vi "GetProperties.vi"(8 "error in":errorcluster, 11 "Decoration in":refnum<class "Decoration.lvclass">) -> (0 "error out":errorcluster, 3 "Decoration out":refnum<class "Decoration.lvclass">)   [LabVIEW 2014, in "Raspberry Pi Compatible Compiler for LabVIEW.lvlib" / "Decoration.lvclass"]
uses:
  Decoration.lvclass
  Decoration.lvclass/Decoration.ctl
  GObject/GObject.lvclass
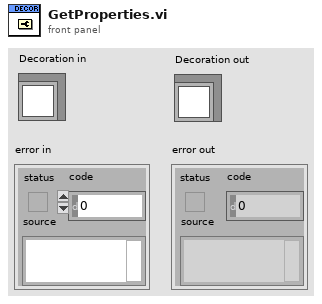
[diagram p1: front panel]
types:
  T1 = typedef "LVForegroundBackgroundColorsTypeDef.ctl" = cluster{"FG Color":u32, "BG Color":u32}
  T2 = typedef "LVBoundsTypeDef.ctl" = cluster{"Width":u32, "Height":u32}
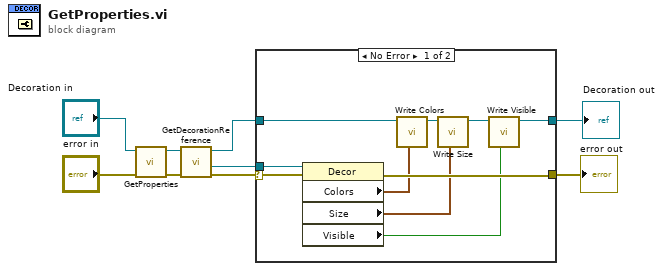
[diagram p0: block diagram]
diagram:
  n1 = call-parent "GetProperties.vi"("error in"="error in", "GObject in"="Decoration in") -> ("error out"=w2:errorcluster, "GObject out"=w4:refnum<class "Decoration.lvclass">)  [unwired: 8 in]
  n2 = call "GetDecorationReference.vi"("error in"=w2, "Decoration in"=w4) -> ("error out"=w6:errorcluster, "Decoration reference"=w5:refnum<vi>, "Decoration out"=w7:refnum<class "Decoration.lvclass">)  [unwired: 7 in]
  n3 = case shown="No Error" w6 {
    selector: w6 -> [w19 w21]
    tunnel: [w17 w21] -> w9
    tunnel: [w10 w20] -> w8
    tunnel: w5 -> [w18 _]
    tunnel: w7 -> [w16 w20]
    frame No Error {
      n4 = property class="Decor"(reference=w18, error in=w19) -> (error out=w17:errorcluster, "Colors"=w15:T1, "Size"=w13:T2, "Visible"=w11:bool)  [unwired: 1 out]
      n5 = call "Write Colors.vi"("Colors"=w15, "Decoration in"=w16) -> ("Decoration out"=w14:refnum<class "Decoration.lvclass">)  [unwired: 7 in]
      n6 = call "Write Size.vi"("Size"=w13, "Decoration in"=w14) -> ("Decoration out"=w12:refnum<class "Decoration.lvclass">)  [unwired: 7 in]
      n7 = call "Write Visible.vi"("Visible"=w11, "Decoration in"=w12) -> ("Decoration out"=w10:refnum<class "Decoration.lvclass">)  [unwired: 7 in]
    }
    frame Error {
    }
  }
  "error out" <- w9
  "Decoration out" <- w8
